vi "Add Item.vi"(8 "error in (no error)":errorcluster, 10 "text":string, 11 "MenueItem in":refnum<class "MenueItem.lvclass">) -> (0 "error out":errorcluster, 3 "MenueItem out":refnum<class "MenueItem.lvclass">)   [LabVIEW 2016, in "MenueItem.lvclass"]
uses:
  MenueItem.lvclass
  System.Windows.Forms
  MenueItem.lvclass/MenueItem.ctl
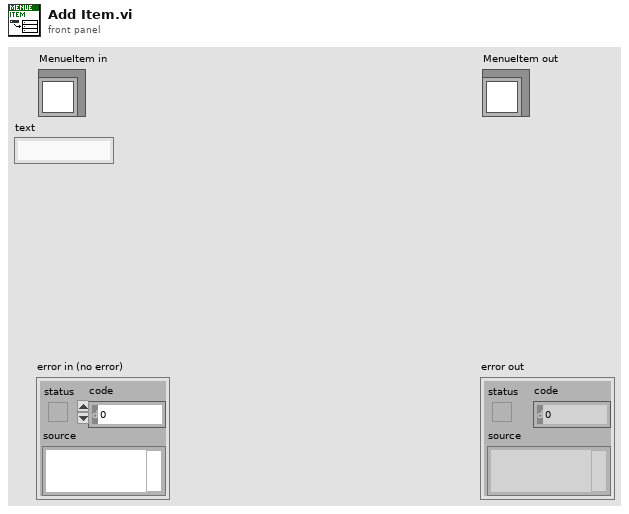
[diagram p1: front panel]
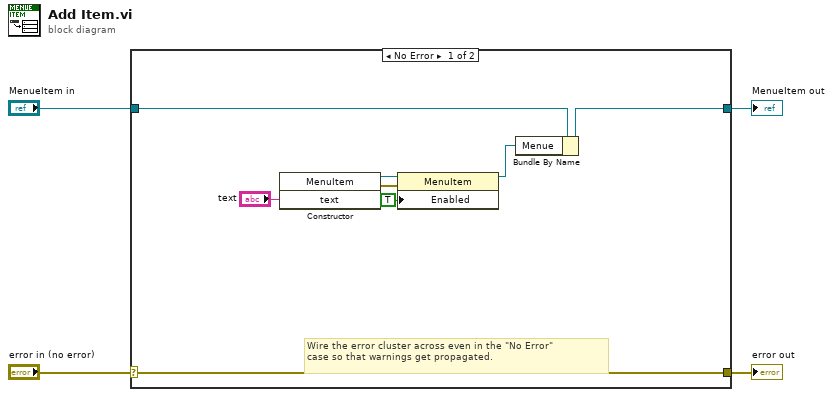
[diagram p0: block diagram]
diagram:
  n1 = case shown="No Error" "error in (no error)" {
    selector: "error in (no error)" -> [w12 w14]
    tunnel: [w12 w14] -> w3
    tunnel: [w5 w13] -> w1
    tunnel: "MenueItem in" -> [w11 w13]
    frame No Error {
      # "Wire the error cluster across even in the \"No Error\"\ncase so that warnings get propagated."
      n2 = constructor class="MenuItem"("text"="text") -> (reference out=w9:refnum<k24>, error out=w8:errorcluster)  [unwired: 3 in, 2 out]
      n3 = property class="MenuItem"(reference=w9, error in=w8, "Enabled"=TRUE) -> (reference out=w6:refnum<k24>)  [unwired: 1 out]
      n4 = Bundle By Name(cluster=w11, "Menue"=w6) -> (w5:refnum<class "MenueItem.lvclass">)
    }
    frame Error {
    }
  }
  "error out" <- w3
  "MenueItem out" <- w1
